vi "Read status reference.vi"(8 "error in (no error)":errorcluster, 11 "SP in":refnum<class "Save messages PGserver.lvclass">) -> (0 "error out":errorcluster, 2 "Status":T1, 3 "SP out":refnum<class "Save messages PGserver.lvclass">)   [LabVIEW 2019, in "Save messages PGserver.lvclass"]
uses:
  Save messages PGserver.lvclass
  Modbus/Eth Status/Ctl/ICPCON Status.ctl
  Modbus/MB_TCP2/MB_TCP_State.ctl
  Save messages PGserver.lvclass/Save messages PGserver.ctl
  Modbus/Eth Status/Eth Status.lvlib
  Modbus/MB_TCP2/MB_TCP.lvclass
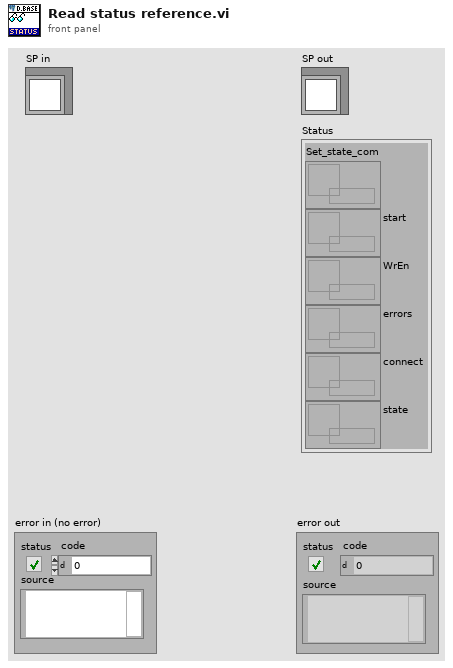
[diagram p1: front panel]
types:
  T1 = typedef "Eth Status.lvlib/ICPCON Status.ctl" = cluster{"Set_state_com":refnum<data-value>, "start":refnum<data-value>, "WrEn":refnum<data-value>, "errors":refnum<data-value>, "connect":refnum<data-value>, "state":refnum<data-value>}
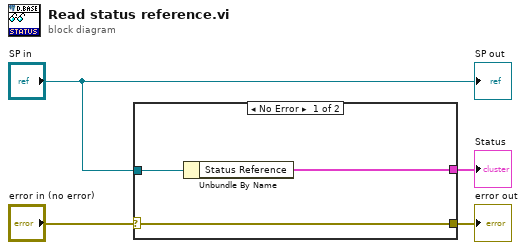
[diagram p0: block diagram]
diagram:
  n1 = case shown="No Error" "error in (no error)" {
    selector: "error in (no error)" -> [w7 w8]
    tunnel: [w7 w8] -> w3
    tunnel: "SP in" -> [w5 _]
    tunnel: [w6 _] -> w2
    frame No Error {
      n2 = Unbundle By Name(w5) -> ("Status Reference"=w6:T1)
    }
    frame Error {
    }
  }
  "error out" <- w3
  "Status" <- w2
  "SP out" <- "SP in"
